vi "OutputTurret.vi"() -> ()   [LabVIEW 2020]
uses:
  <vilib>/Rock Robotics/WPI/ThirdParty/Phoenix-LabVIEW/Motor Controller/Controls/CTRE_Phoenix_MotorControl_ControlMode.ctl
  refnumbers.vi
  GRNF_CTREMotor.vi
  robotoutputs.vi
  sensordata.vi
  driverdata.vi
  robotconstants.vi
  TAI_Motor.vi
  <vilib>/Rock Robotics/WPI/ThirdParty/Phoenix-LabVIEW/Motor Controller/Get/CTRE_Phoenix_MotorController_GetSelectedSensorData.vi
panel:
  in  "Arbitrary Feed Forward [-1,1]":dbl
  in  "S-Curve Strength":i32=4
  out "Turret Position and Velocity":cluster{dbl, "f":dbl, dbl}(graph)
  out "Position":dbl
  in  "PID Parameters":T1={"Kp"=0.3, "Ki"=0.0005, "Kd"=0.0, "Kf (don't use)"=0.0, "I-Zone"=10.0} {"Kd" min=0.0; "Ki" min=0.0; "Kp" min=0.0}
  in  "Acceleration (deg/s^2)":i32=10000
  in  "Cruise Velocity (deg/s)":i32=350
  in  "Plotting":bool
  in  "Manual Override Turret":bool
  in  "Turret Command (deg)":dbl
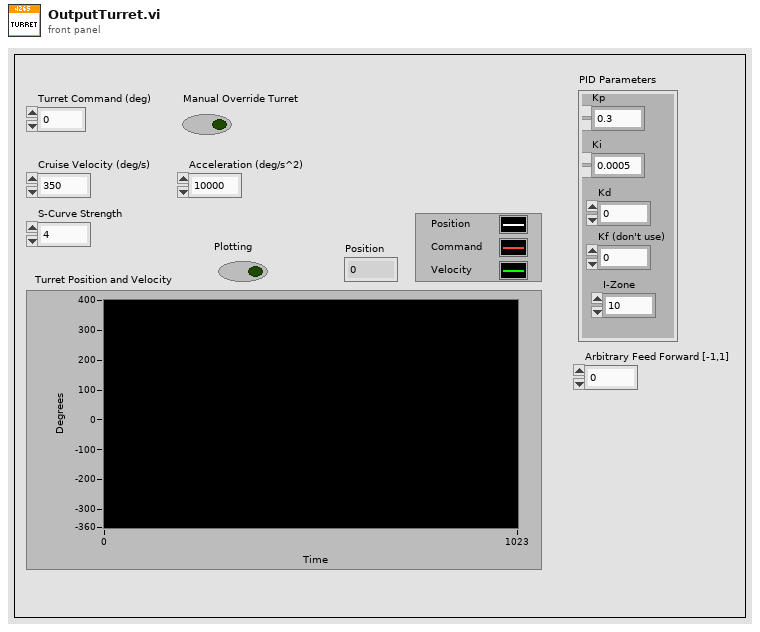
[diagram p1: front panel]
types:
  T1 = cluster{"Kp":dbl, "Ki":dbl, "Kd":dbl, "Kf (don't use)":dbl, "I-Zone":dbl}
  T2 = enum16{"DemandType_Neutral", "DemandType_AuxPID", "DemandType_ArbitraryFeedForward"}
  T3 = cluster{"Cruise Velocity (deg/s)":i32, "Acceleration (deg/s^2)":i32, "S-Curve Strength":i32}
  T4 = typedef "WPI_MotorControlDeviceRef.ctl" = cluster{"DeviceStatus":errorcluster, "Type":T5, "PWM":cluster{"PWM Channel":T6, "DeadBand":T7}, "CAN":cluster{"Device Number":u8, "SetOutput VI Ref":variant, "GetOutput VI Ref":variant, "Enable VI Ref":variant, "Disable VI Ref":variant, "Data":variant}, "Invert":bool, "DIO PWM":cluster{"PWM \"Enable\" Channel":T6, "DIOChannel":T8, "PWM Rate":dbl}}
  T5 = typedef "WPI_MotorControlType.ctl" = enum16{"PWM", "CAN", "DIO PWM"}
  T6 = typedef "FPGA_DIOPWMChannel.ctl" = enum8{"PWM 0", "PWM 1", "PWM 2", "PWM 3", "PWM 4", "PWM 5", "PWM 6", "PWM 7", "PWM 8", "PWM 9", "PWM MXP 0", "PWM MXP 1", "PWM MXP 2", "PWM MXP 3", "PWM MXP 4", "PWM MXP 5", "PWM MXP 6", "PWM MXP 7", "PWM MXP 8", "PWM MXP 9", "Invalid"}
  T7 = typedef "WPI_PWMDeadband.ctl" = cluster{"Name":string, "maxPositivePwm":i32, "minPositivePwm":i32, "centerPwm":i32, "maxNegativePwm":i32, "minNegativePwm":i32, "angularRange":u16}
  T8 = typedef "FPGA_DIOChannel.ctl" = enum8{"DIO 0", "DIO 1", "DIO 2", "DIO 3", "DIO 4", "DIO 5", "DIO 6", "DIO 7", "DIO 8", "DIO 9", "DIO MXP 0", "DIO MXP 1", "DIO MXP 2", "DIO MXP 3", "DIO MXP 4", "DIO MXP 5", "DIO MXP 6", "DIO MXP 7", "DIO MXP 8", "DIO MXP 9", "DIO MXP 10", "DIO MXP 11", "DIO MXP 12", "DIO MXP 13", "DIO MXP 14", "DIO MXP 15", "SPI Port CS1", "SPI Port CS2", "SPI Port CS3", "SPI Port MISO", "SPI Port MOSI", "Invalid"}
  T9 = cluster{"Cruise Velocity (deg/s)":bool, "Acceleration (deg/s^2)":bool, "S-Curve Strength":bool}
  T10 = cluster{"Kp":bool, "Ki":bool, "Kd":bool, "Kf (don't use)":bool, "I-Zone":bool}
  T11 = typedef "CTRE_Phoenix_MotorControl_ControlMode.ctl" = u16
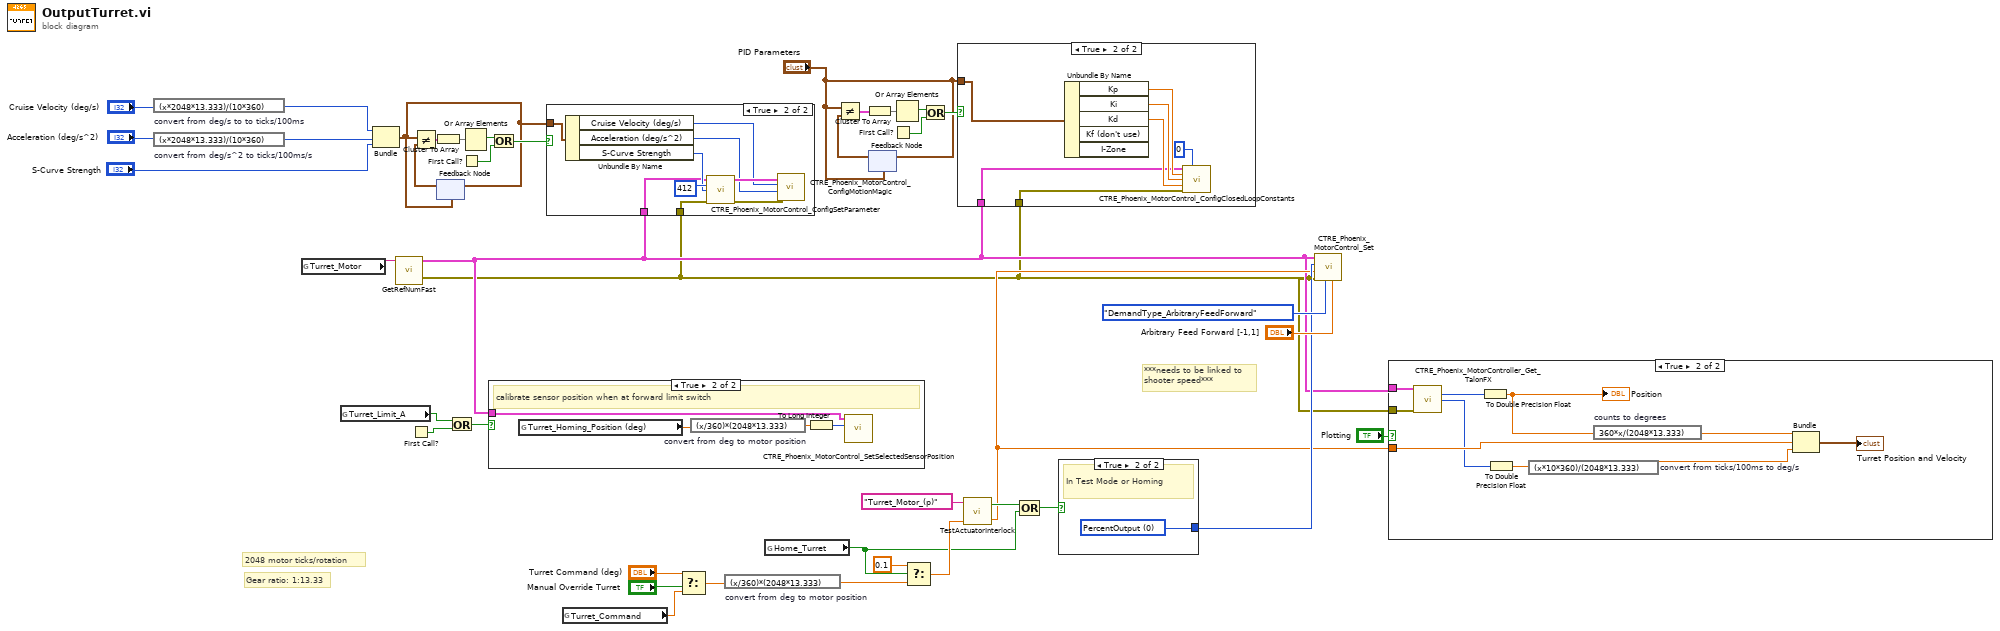
[diagram p0: block diagram]
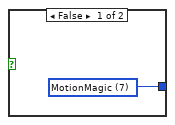
[diagram p4: hidden frame]
diagram:
  # "***needs to be linked to\nshooter speed***"
  # "Gear ratio: 1:13.33"
  # "2048 motor ticks/rotation"
  n1 = expression code="(x*2048*13.333)/(10*360)" "convert from deg/s to to ticks/100ms"("Cruise Velocity (deg/s)") -> (w15:i32)
  n2 = expression code="(x*2048*13.333)/(10*360)" "convert from deg/s^2 to ticks/100ms/s"("Acceleration (deg/s^2)") -> (w14:i32)
  n3 = global read "refnumbers.vi" "Turret_Motor"() -> (w40:string)
  n4 = global read "sensordata.vi" "Turret_Limit_A"() -> (w2:bool)
  n5 = Bundle("Cruise Velocity (deg/s)"=w15, "Acceleration (deg/s^2)"=w14, "S-Curve Strength"="S-Curve Strength") -> (w6:T3)  [unwired: 1 in]
  n6 = call-poly "GetRefNumFast.vi"("RefNum Name"=w40) -> ("Error"=w4:errorcluster, "Device Reference"=w5:T4)  [unwired: 5 in]
  n7 = First Call?() -> (First Call?: T/F=w1:bool)
  n8 = feedback #1(w6) -> (w7:T3)
  n9 = Not Equal?(x=w6, y=w7) -> (x != y?=w10:T9)
  n10 = Cluster To Array(cluster=w10) -> (array=w9:bool[])
  n11 = feedback-in #1(w6) -> ()
  n12 = Or(x=w2, y=w1) -> (x .or. y?=w3:bool)
  n13 = First Call?() -> (First Call?: T/F=w12:bool)
  n14 = Or Array Elements(Boolean array=w9) -> (logical OR=w11:bool)
  n15 = case shown="True" w3 {
    tunnel: w5 -> [_ w43]
    frame False {
    }
    frame True {
      # "calibrate sensor position when at forward limit switch"
      n16 = global read "robotconstants.vi" "Turret_Homing_Position (deg)"() -> (w42:dbl)
      n17 = expression code="(x/360)*(2048*13.333)" "convert from deg to motor position"(w42) -> (w45:dbl)
      n18 = To Long Integer(number=w45) -> (32bit integer=w44:i32)
      n19 = call <vilib>:"CTRE_Phoenix_MotorControl_SetSelectedSensorPosition.vi"("New Sensor Position"=w44, "PhoenixMotorControlDevRef"=w43) -> ()  [unwired: 8 in, 2 out]
    }
  }
  n20 = Or(x=w11, y=w12) -> (x .or. y?=w8:bool)
  n21 = case shown="True" w8 {
    tunnel: w6 -> [_ w51]
    tunnel: w5 -> [_ w47]
    tunnel: w4 -> [_ w46]
    frame False {
    }
    frame True {
      n22 = Unbundle By Name(w51) -> ("Cruise Velocity (deg/s)"=w48:i32, "Acceleration (deg/s^2)"=w49:i32, "S-Curve Strength"=w50:i32)
      n23 = call <vilib>:"CTRE_Phoenix_MotorControl_ConfigSetParameter.vi"("PhoenixMotorControlDevRef"=w47, "Parameter"=412 ("New Sensor Position"), "value"=w50, "error in (no error)"=w46) -> ("PhoenixMotorControlDevRef"=w53:T4, "error out"=w52:errorcluster)  [unwired: 10 in]
      n24 = call <vilib>:"CTRE_Phoenix_MotorControl_ConfigMotionMagic.vi"("error in (no error)"=w52, "Acceleration"=w49, "Cruise Velocity"=w48, "PhoenixMotorControlDevRef"=w53) -> ()  [unwired: 6 in, 2 out]
    }
  }
  n25 = global read "robotoutputs.vi" "Turret_Command"() -> (w25:dbl)
  n26 = Select(t="Turret Command (deg)", s="Manual Override Turret", f=w25) -> (s? t:f=w34:dbl)
  n27 = expression code="(x/360)*(2048*13.333)" "convert from deg to motor position"(w34) -> (w26:dbl)
  n28 = global read "driverdata.vi" "Home_Turret"() -> (w23:bool)
  n29 = feedback #2("PID Parameters") -> (w17:T1)
  n30 = Not Equal?(x="PID Parameters", y=w17) -> (x != y?=w20:T10)
  n31 = Cluster To Array(cluster=w20) -> (array=w19:bool[])
  n32 = feedback-in #2("PID Parameters") -> ()
  n33 = First Call?() -> (First Call?: T/F=w22:bool)
  n34 = Or Array Elements(Boolean array=w19) -> (logical OR=w21:bool)
  n35 = Select(t=0.1, s=w23, f=w26) -> (s? t:f=w27:dbl)
  n36 = Or(x=w21, y=w22) -> (x .or. y?=w18:bool)
  n37 = case shown="True" w18 {
    tunnel: w5 -> [_ w57]
    tunnel: w4 -> [_ w56]
    tunnel: "PID Parameters" -> [_ w55]
    frame False {
    }
    frame True {
      n38 = Unbundle By Name(w55) -> ("Kp"=w59:dbl, "Ki"=w60:dbl, "Kd"=w61:dbl)  [unwired: 2 out]
      n39 = call <vilib>:"CTRE_Phoenix_MotorControl_ConfigClosedLoopConstants.vi"("PhoenixMotorControlDevRef"=w57, "slotIdx"=0, "P"=w59, "I"=w60, "D"=w61, "error in (no error)"=w56) -> ()  [unwired: 8 in, 2 out]
    }
  }
  n40 = call-poly "TestActuatorInterlock.vi"("Normal Output"=w27, "Actuator Name"="Turret_Motor_(p)" ("Actuator_Name")) -> ("Interlock Output"=w24:dbl, "Testing This Actuator"=w30:bool)  [unwired: 1 in]
  n41 = Compound Arithmetic op=OR(w30, w23) -> (w29:bool)
  n42 = case shown="True" w29 {
    tunnel: [w62 w63] -> w31
    frame False {
      w62 = T11 7 items=["PercentOutput"=0, "Position"=1, "Velocity"=2, "Current"=3, "Follower"=5, "MotionProfile"=6, "MotionMagic"=7, "MotionProfileArc"=10, "Disabled"=15] ("f")
    }
    frame True {
      w63 = T11 0 items=["PercentOutput"=0, "Position"=1, "Velocity"=2, "Current"=3, "Follower"=5, "MotionProfile"=6, "MotionMagic"=7, "MotionProfileArc"=10, "Disabled"=15] ("Control Mode")
      # "In Test Mode or Homing"
    }
  }
  n43 = call <vilib>:"CTRE_Phoenix_MotorControl_Set.vi"("Demand1"="Arbitrary Feed Forward [-1,1]", "DemandType"=T2."DemandType_ArbitraryFeedForward", "error in (no error)"=w4, "Output"=w24, "Control Mode"=w31, "PhoenixMotorControlDevRef"=w5) -> ()  [unwired: 4 in, 2 out]
  n44 = case shown="True" "Plotting" {
    tunnel: w24 -> [_ w73]
    tunnel: w4 -> [_ w65]
    tunnel: w5 -> [_ w64]
    frame False {
    }
    frame True {
      n45 = call-poly <vilib>:"CTRE_Phoenix_MotorController_Get_TalonFX.vi"("PhoenixMotorControlDevRef"=w64, "error in"=w65) -> ("Position (Raw Sensor Units)"=w69:i32, "Velocity (Raw Sensor Units per 100 ms)"=w70:i32)  [unwired: 10 in, 2 out]
      n46 = To Double Precision Float(number=w69) -> (double precision float=w68:dbl)
      "Position" <- w68
      n47 = To Double Precision Float(number=w70) -> (double precision float=w71:dbl)
      n48 = expression code="(x*10*360)/(2048*13.333)" "convert from ticks/100ms to deg/s"(w71) -> (w72:dbl)
      n49 = expression code="360*x/(2048*13.333)" "counts to degrees"(w68) -> (w67:dbl)
      n50 = Bundle(w67, "Interlock Output"=w73, w72) -> (→"Turret Position and Velocity":cluster{dbl, "Interlock Output":dbl, dbl})  [unwired: 1 in]
    }
  }
